vi "Get Test ID.vi"(8 "error in":errorcluster, 11 "Test In":refnum<class>) -> (0 "error out":errorcluster, 1 "IsTestCase":bool, 2 "id":string, 3 "Test Out":refnum<class>, 5 "GUID":string)   [LabVIEW 2011, in "GraphicalTestRunner.lvlib"]
uses:
  GraphicalTestRunner.lvlib
  Classes/TestCase/TestCase.lvclass
  Classes/TestSuite/TestSuite.lvclass
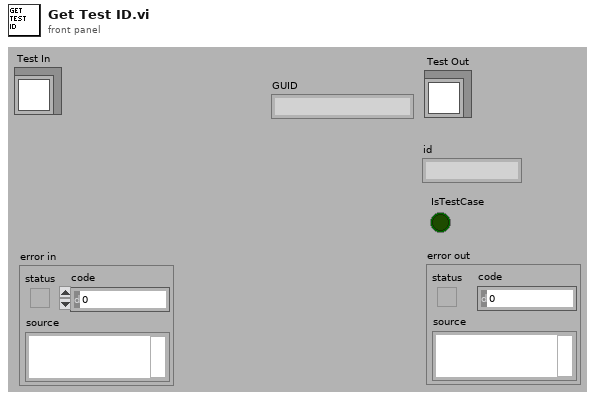
[diagram p1: front panel]
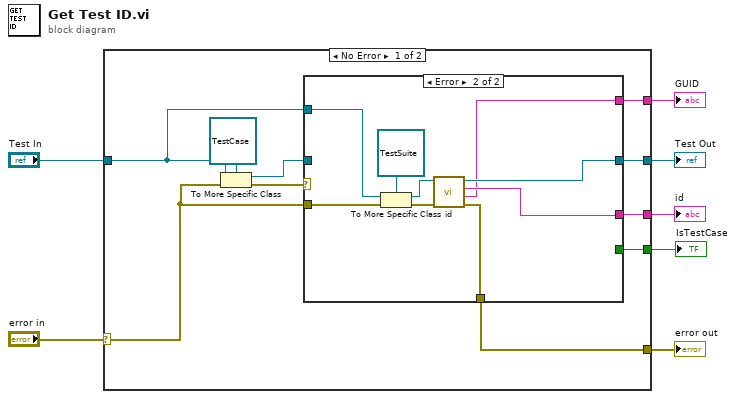
[diagram p0: block diagram]
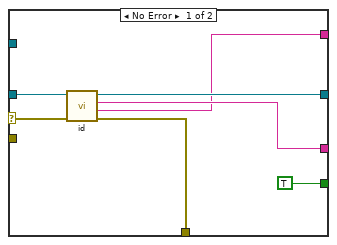
[diagram p2: hidden frame]
diagram:
  n1 = case shown="No Error" "error in" {
    selector: "error in" -> [w10 w35]
    tunnel: [w17 w35] -> w7
    tunnel: [w16 w34] -> w6
    tunnel: [w15 _] -> w5
    tunnel: "Test In" -> [w11 w34]
    tunnel: [w9 _] -> w2
    tunnel: [w8 _] -> w1
    frame No Error {
      n2 = To More Specific Class(target class=refnum<class "TestCase.lvclass"> refnum ("TestCase.lvclass"), reference=w11, error in=w10) -> (specific class reference=w13:refnum<class "TestCase.lvclass">, error out=w14:errorcluster)
      n3 = case shown="Error" w14 {
        selector: w14 -> [w20 _]
        tunnel: [w24 w26] -> w17
        tunnel: [w23 w27] -> w16
        tunnel: [w22 w28] -> w15
        tunnel: w13 -> [w21 _]
        tunnel: w10 -> [_ w32]
        tunnel: w11 -> [_ w31]
        tunnel: [TRUE ("IsTestCase") _] -> w9
        tunnel: [w18 w25] -> w8
        frame No Error {
          n4 = call-dynamic "id.vi"("error in (no error)"=w20, "TestCase in"=w21) -> ("error out"=w24:errorcluster, "GUID"=w18:string, "id"=w22:string, "TestCase out"=w23:refnum<class "TestCase.lvclass">)  [unwired: 6 in]
        }
        frame Error {
          n5 = To More Specific Class(target class=refnum<class "TestSuite.lvclass"> refnum ("TestSuite.lvclass"), reference=w31, error in=w32) -> (specific class reference=w29:refnum<class "TestSuite.lvclass">, error out=w30:errorcluster)
          n6 = call-dynamic "id.vi"("error in (no error)"=w30, "TestSuite in"=w29) -> ("error out"=w26:errorcluster, "GUID"=w25:string, "Description"=w28:string, "TestSuite out"=w27:refnum<class "TestSuite.lvclass">)  [unwired: 6 in]
        }
      }
    }
    frame Error {
    }
  }
  "error out" <- w7
  "Test Out" <- w6
  "id" <- w5
  "IsTestCase" <- w2
  "GUID" <- w1
